vi "Motor Set Power.vi"(8 "error in":errorcluster, 9 "Linear Response":bool, 10 "Output":dbl, 11 "Motor In":T1={"MotorControlDeviceRef"={"DeviceStatus"={"status"=FALSE, "code"=0, "source"=""}, "Type"=enum."PWM", "PWM"={"Controller"=enum."Controller 1", "PWM Channel"=enum."Invalid", "DeadBand"={"Name"="", "maxPositivePwm"=0, "minPositivePwm"=0, "centerPwm"=0, "maxNegativePwm"=0, "minNegativePwm"=0, "angularRange"=0}}, "CAN"={"Device Number"=0, "Control Mode"=enum."Percent VBus", "Semaphore"=refnum, "Max Vout"=12.0, "TalonSRX Control Mode"=enum."Percent VBus"}, "Invert"=FALSE, "TransformRef"=refnum, "InvTransformRef"=refnum}, "Last Motor Power"=0.0}) -> (0 "error out":errorcluster, 3 "Motor Out":T1={"MotorControlDeviceRef"={"DeviceStatus"={"status"=FALSE, "code"=0, "source"=""}, "Type"=enum."PWM", "PWM"={"Controller"=enum."Controller 1", "PWM Channel"=enum."Invalid", "DeadBand"={"Name"="", "maxPositivePwm"=0, "minPositivePwm"=0, "centerPwm"=0, "maxNegativePwm"=0, "minNegativePwm"=0, "angularRange"=0}}, "CAN"={"Device Number"=0, "Control Mode"=enum."Percent VBus", "Semaphore"=refnum, "Max Vout"=12.0, "TalonSRX Control Mode"=enum."Percent VBus"}, "Invert"=FALSE, "TransformRef"=refnum, "InvTransformRef"=refnum}, "Last Motor Power"=0.0})   [LabVIEW 2014]
uses:
  Motor Typedef.ctl
  <vilib>/Rock Robotics/WPI/MotorControl/WPI_MotorControlDeviceRef.ctl
  <vilib>/Rock Robotics/WPI/MotorControl/WPI_MotorControlType.ctl
  <vilib>/Rock Robotics/SystemInterfaces/Typedef/FPGA_TypedefDigitalModule.ctl
  <vilib>/Rock Robotics/SystemInterfaces/DIO/FPGA_DIOPWMChannel.ctl
  <vilib>/Rock Robotics/WPI/PWM/WPI_PWMDeadband.ctl
  <vilib>/Rock Robotics/WPI/CAN/Jaguar/SubVIs/WPI_CANJaguar_ControlMode.ctl
  <vilib>/Rock Robotics/WPI/CAN/TalonSRX/WPI_CANTalonSRX_APIControlMode.ctl
  <vilib>/Rock Robotics/WPI/PWM/WPI_PWMTransform_ConPane.ctl
  Global Objects.vi
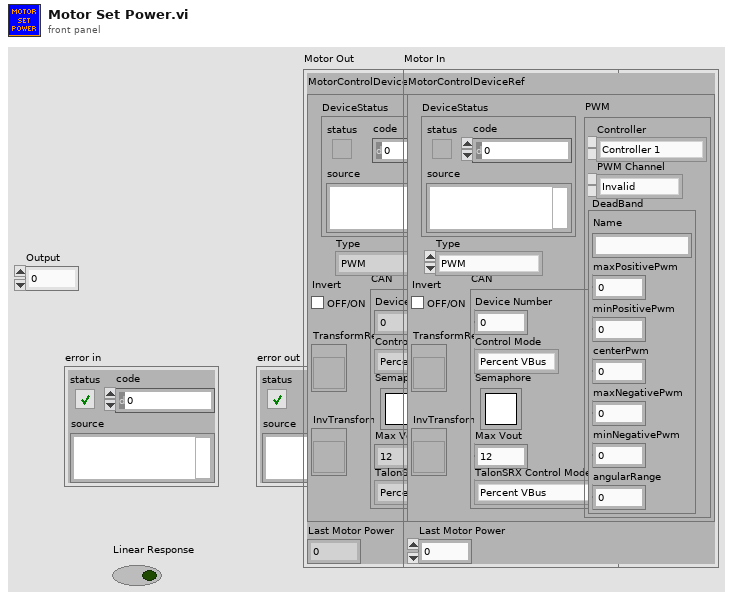
[diagram p1: front panel]
types:
  T1 = typedef "Motor Typedef.ctl" = cluster{"MotorControlDeviceRef":T2, "Last Motor Power":dbl}
  T2 = typedef "WPI_MotorControlDeviceRef.ctl" = cluster{"DeviceStatus":errorcluster, "Type":T3, "PWM":cluster{"Controller":T4, "PWM Channel":T5, "DeadBand":T6}, "CAN":cluster{"Device Number":u8, "Control Mode":T7, "Semaphore":T8, "Max Vout":dbl, "TalonSRX Control Mode":T9}, "Invert":bool, "TransformRef":T10, "InvTransformRef":T10}
  T3 = typedef "WPI_MotorControlType.ctl" = enum16{"PWM", "CAN", "CANTalonSRX"}
  T4 = typedef "FPGA_TypedefDigitalModule.ctl" = enum16{"Controller 1"}
  T5 = typedef "FPGA_DIOPWMChannel.ctl" = enum8{"PWM 0", "PWM 1", "PWM 2", "PWM 3", "PWM 4", "PWM 5", "PWM 6", "PWM 7", "PWM 8", "PWM 9", "PWM MXP 0", "PWM MXP 1", "PWM MXP 2", "PWM MXP 3", "PWM MXP 4", "PWM MXP 5", "PWM MXP 6", "PWM MXP 7", "PWM MXP 8", "PWM MXP 9", "Invalid"}
  T6 = typedef "WPI_PWMDeadband.ctl" = cluster{"Name":string, "maxPositivePwm":i32, "minPositivePwm":i32, "centerPwm":i32, "maxNegativePwm":i32, "minNegativePwm":i32, "angularRange":u16}
  T7 = typedef "WPI_CANJaguar_ControlMode.ctl" = enum8{"Percent VBus", "Current", "Speed", "Position", "Voltage"}
  T8 = typedef "Semaphore RefNum" = refnum<k1>
  T9 = typedef "WPI_CANTalonSRX_APIControlMode.ctl" = enum8{"Percent VBus", "Speed", "Position", "Slave", "Unchanged / Invalid"}
  T10 = typedef "WPI_PWMTransform_ConPane.ctl" = refnum<vi>
  T11 = typedef "Configuration.ctl" = cluster{"Throttle Dead Zone":dbl, "Throttle Ramp Rate":dbl, "Turn Dead Zone":dbl, "Auton":cluster{"Motion Plan P":dbl, "Motion Plan I":dbl, "Motion Plan D":dbl}, "Auto Upshift Enabled":bool, "Upshift Min Throttle":dbl, "Upshift Min Velocity":dbl, "Min time between shifts":dbl}
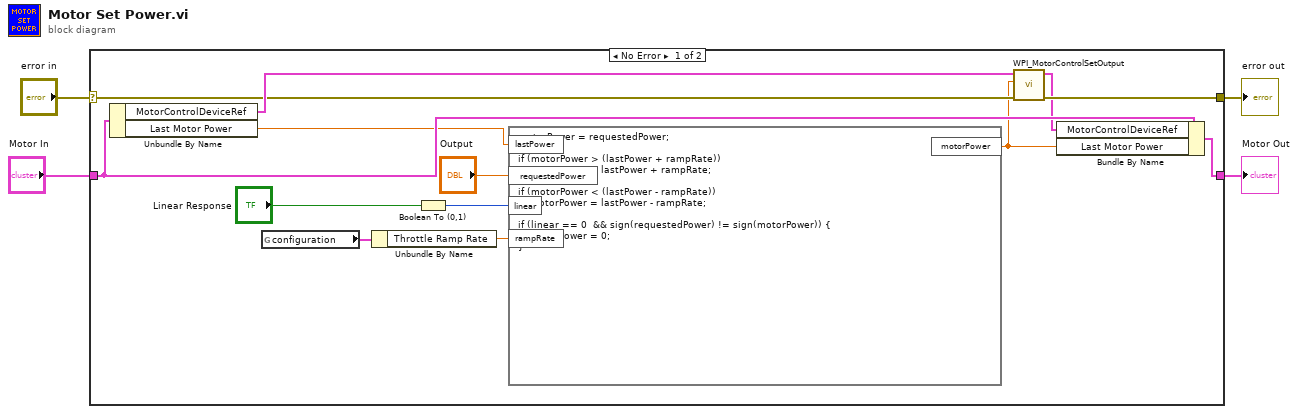
[diagram p0: block diagram]
diagram:
  n1 = case shown="No Error" "error in" {
    selector: "error in" -> [w16 w19]
    tunnel: [w15 w19] -> w3
    tunnel: "Motor In" -> [w14 w18]
    tunnel: [w12 w18] -> w1
    frame No Error {
      n2 = Unbundle By Name(w14) -> ("MotorControlDeviceRef"=w17:T2, "Last Motor Power"=w7:dbl)
      n3 = global read "Global Objects.vi" "configuration"() -> (w11:T11)
      n4 = Unbundle By Name(w11) -> ("Throttle Ramp Rate"=w6:dbl)
      n5 = Boolean To (0,1)(Boolean="Linear Response") -> (0, 1=w9:i16)
      n6 = formula code="motorPower = requestedPower;\n\nif (motorPower > (lastPower + rampRate))\n    motorPower = lastPower + rampRate;\n\nif (motorPower < (lastPower - rampRate))\n    motorPower = lastPower - rampRate;\n\nif (linear == 0  && sign(requestedPower) != sign(motorPower)) {\n    motorPower = 0;\n}"("lastPower"=w7, "requestedPower"="Output", "linear"=w9, "rampRate"=w6) -> ("motorPower"=w8:dbl)
      n7 = call <vilib>:"WPI_MotorControlSetOutput.vi"("error in (no error)"=w16, "Output"=w8, "MotorControlDevRef"=w17) -> ("error out"=w15:errorcluster, "MotorControlDevRef"=w13:T2)  [unwired: 6 in, 1 out]
      n8 = Bundle By Name(cluster=w14, "MotorControlDeviceRef"=w13, "Last Motor Power"=w8) -> (w12:T1)
    }
    frame Error {
    }
  }
  "error out" <- w3
  "Motor Out" <- w1
